vi "set_main_panel.vi"(6 "Active Element":refnum<vi>, 8 "Working Directory":refnum<vi>, 9 "Simulation Log":refnum<vi>, 10 "Plant Structure":refnum<vi>, 11 "Iteration":refnum<vi>) -> ()   [LabVIEW 2019]
uses:
  lib/libSimulationControl/libSimulationControl.lvlib
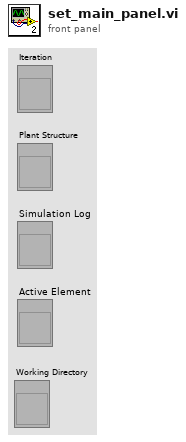
[diagram p1: front panel]
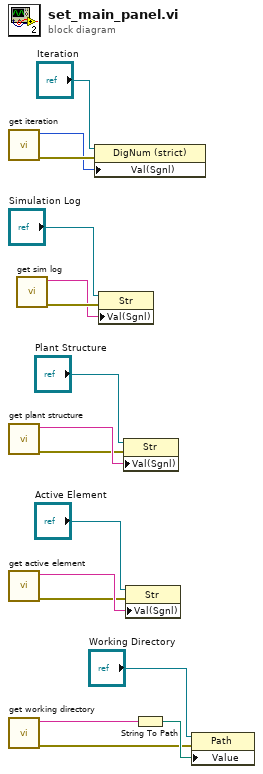
[diagram p0: block diagram]
diagram:
  n1 = call "get iteration.vi"() -> ("error out"=w2:errorcluster, "function return"=w1:i32)  [unwired: 10 in]
  n2 = call "get plant structure.vi"() -> ("error out"=w5:errorcluster, "function return"=w6:string)  [unwired: 10 in]
  n3 = call "get active element.vi"() -> ("error out"=w8:errorcluster, "active_element"=w9:string)  [unwired: 10 in]
  n4 = call "get working directory.vi"() -> ("error out"=w7:errorcluster, "function return"=w10:string)  [unwired: 10 in]
  n5 = call "get sim log.vi"() -> ("error out"=w4:errorcluster, "function return"=w3:string)  [unwired: 10 in]
  n6 = property on="Property Node" class="DigNum (strict)"(reference="Iteration", error in=w2, "Val(Sgnl)"=w1) -> ()  [unwired: 2 out]
  n7 = property on="Property Node" class="Str"(reference="Simulation Log", error in=w4, "Val(Sgnl)"=w3) -> ()  [unwired: 2 out]
  n8 = property on="Property Node" class="Str"(reference="Plant Structure", error in=w5, "Val(Sgnl)"=w6) -> ()  [unwired: 2 out]
  n9 = property on="Property Node" class="Str"(reference="Active Element", error in=w8, "Val(Sgnl)"=w9) -> ()  [unwired: 2 out]
  n10 = String To Path(string=w10) -> (path=w11:path)
  n11 = property on="Property Node" class="Path"(reference="Working Directory", error in=w7, "Value"=w11) -> ()  [unwired: 2 out]
